vi "Countdown.vi"(2 "Time / ms":dbl, 3 "notifier in":refnum<notifier>) -> ()   [LabVIEW 2017, in "GP22_TDC_Arduinoed.lvlib"]
uses:
  GP22_TDC_Arduinoed.lvlib
panel:
  out "Gauge":dbl(knob) scale=0.0..100.0
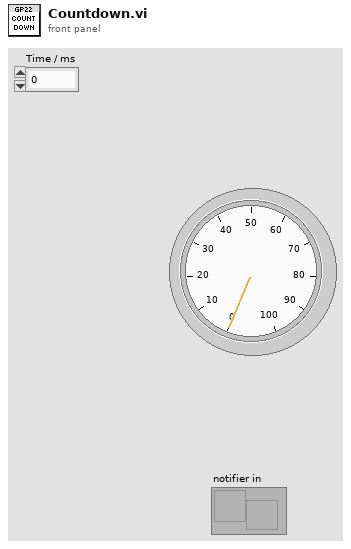
[diagram p1: front panel]
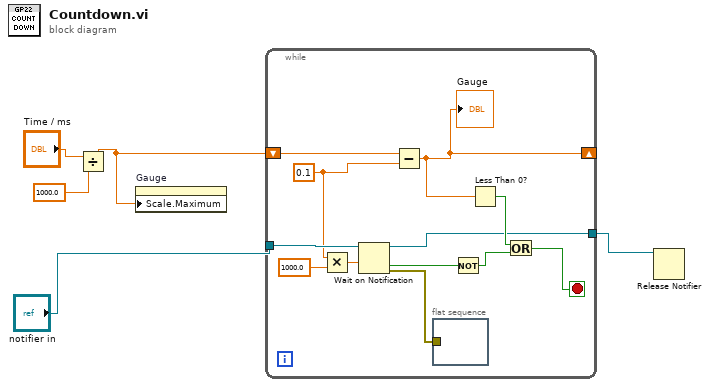
[diagram p0: block diagram]
diagram:
  n1 = Divide(x="Time / ms", y=1000.0) -> (x/y=w4:dbl)
  n2 = property on="Gauge" class="Knob (strict)"("Scale.Maximum"=w4) -> ()  [unwired: 2 in, 2 out]
  n3 = while {
    shift-right: [w16] -> _
    shift-left: w4 -> [w17]
    tunnel: "notifier in" -> [w14]
    tunnel: [w11] -> w1
    stop <- w13 stop-if-true
    w9 = 0.1 ("Period")
    n4 = Multiply(x=w9, y=1000.0) -> (x*y=w10:dbl)
    n5 = Wait on Notification(notifier=w14, timeout in ms (-1)=w10) -> (notifier out=w11:refnum<notifier>, timed out?=w7:bool, error out=w12:errorcluster)  [unwired: 2 in, 1 out]
    n6 = Subtract(x=w17, y=w9) -> (x-y=w16:dbl)
    "Gauge" <- w16
    n7 = flat-sequence {
      tunnel: w12 -> [_]
      frame #0 {
      }
    }
    n8 = Not(x=w7) -> (.not. x?=w6:bool)
    n9 = Less Than 0?(x=w16) -> (x < 0?=w15:bool)
    n10 = Or(x=w15, y=w6) -> (x .or. y?=w13:bool)
  }
  n11 = Release Notifier(notifier=w1) -> ()  [unwired: 2 in, 3 out]
